vi "Set Front Panel size.vi"(8 "error in (no error)":errorcluster, 11 "VI in":refnum<vi>) -> (0 "error out":errorcluster)   [LabVIEW 2020, in "Execution UI.lvclass"]
uses:
  Execution UI.lvclass
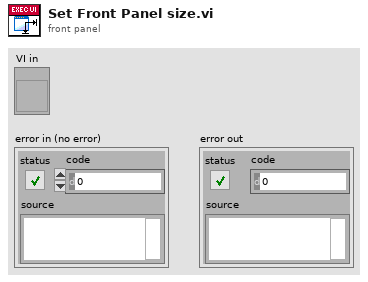
[diagram p1: front panel]
types:
  T1 = typedef "LVRectTypeDef.ctl" = cluster{"Left":i16, "Top":i16, "Right":i16, "Bottom":i16}
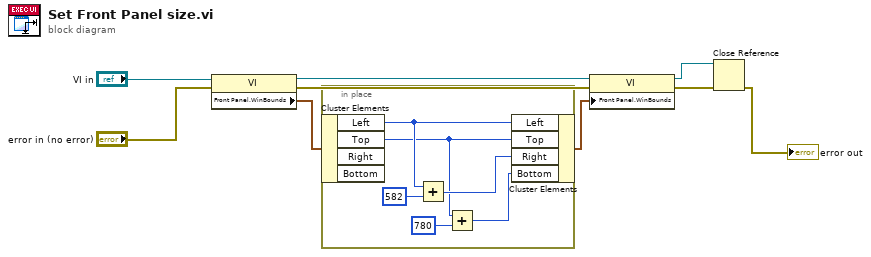
[diagram p0: block diagram]
diagram:
  n1 = property class="VI"(reference="VI in", error in="error in (no error)") -> (reference out=w7:refnum<vi>, error out=w6:errorcluster, "Front Panel.WinBounds"=w4:T1)
  n2 = in-place {
    n3 = in-place-cluster #1(w4) -> ("Left"=w15:i16, "Top"=w11:i16)  [unwired: 2 out]
    n4 = Add(x=w15, y=i16 582) -> (x+y=w13:i16)
    n5 = Add(x=w11, y=i16 780) -> (x+y=w10:i16)
    n6 = in-place-cluster #1("Left"=w15, "Top"=w11, "Right"=w13, "Bottom"=w10) -> (w3:T1)
  }
  n7 = property class="VI"(reference=w7, error in=w6, "Front Panel.WinBounds"=w3) -> (reference out=w5:refnum<vi>, error out=w9:errorcluster)
  n8 = Close Reference(reference=w5, error in (no error)=w9) -> (error out=→"error out":errorcluster)
